vi "ep_Check Array Size.vi"(7 "reset? (F)":bool, 8 "error in (no error)":errorcluster, 11 "number of channels":i32) -> (0 "error out":errorcluster, 3 "number of 3 phases":i32)   [LabVIEW 2014, in "NI_EP_Motor Monitoring.lvlib"]
uses:
  <vilib>/addons/Electrical Power/Motor Monitoring/NI_EP_Motor Monitoring.lvlib
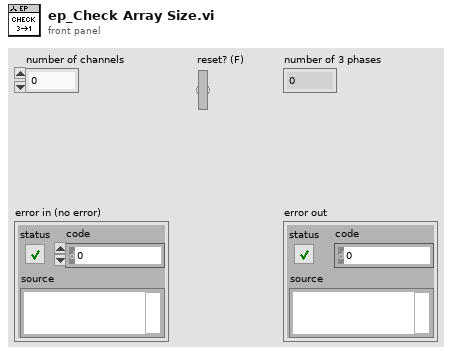
[diagram p1: front panel]
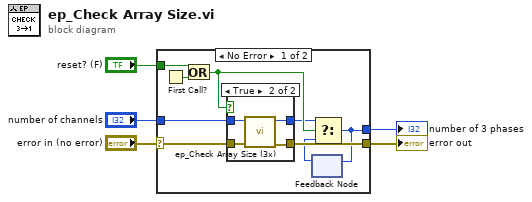
[diagram p0: block diagram]
diagram:
  n1 = case shown="No Error" "error in (no error)" {
    selector: "error in (no error)" -> [w14 w20]
    tunnel: [w13 w20] -> w4
    tunnel: "number of channels" -> [w12 _]
    tunnel: [w9 _] -> w2
    tunnel: "reset? (F)" -> [w10 _]
    frame No Error {
      n2 = First Call?() -> (First Call?: T/F=w11:bool)
      n3 = Or(x=w10, y=w11) -> (x .or. y?=w8:bool)
      n4 = case shown="True" w8 {
        tunnel: w14 -> [w15 w18]
        tunnel: [w15 w17] -> w13
        tunnel: w12 -> [_ w19]
        tunnel: [_ w16] -> w6
        frame False {
        }
        frame True {
          n5 = call <vilib>:"ep_Check Array Size (3x).vi"("error in (no error)"=w18, "number of channels"=w19) -> ("error out"=w17:errorcluster, "number of 3 phases"=w16:i32)  [unwired: 8 in]
        }
      }
      n6 = feedback #1() -> (w7:i32)  [unwired: 1 in]
      n7 = Select(t=w6, s=w8, f=w7) -> (s? t:f=w9:i32)
      n8 = feedback-in #1(w9) -> ()
    }
    frame Error {
    }
  }
  "error out" <- w4
  "number of 3 phases" <- w2
